vi "main.vi"() -> ()   [LabVIEW 2016]
uses:
  controls/Level2.ctl
panel:
  in  "BigCluster":T2
  in  "Cluster":T3
  in  "String":string
  in  "Boolean":bool
  in  "Numeric":dbl
  in  "Tab Control":enum32{"Page 1", "Page SubPanel"}(tab)
  in  "BigCluster":T2
  in  "Cluster":T3
  in  "String":string
  in  "Boolean":bool
  in  "Numeric":dbl
  in  "Panel Name":string
  in  "Refresh":bool
  in  "Listbox":i32(listbox)
  in  "OK":bool
  in  "Stop":bool
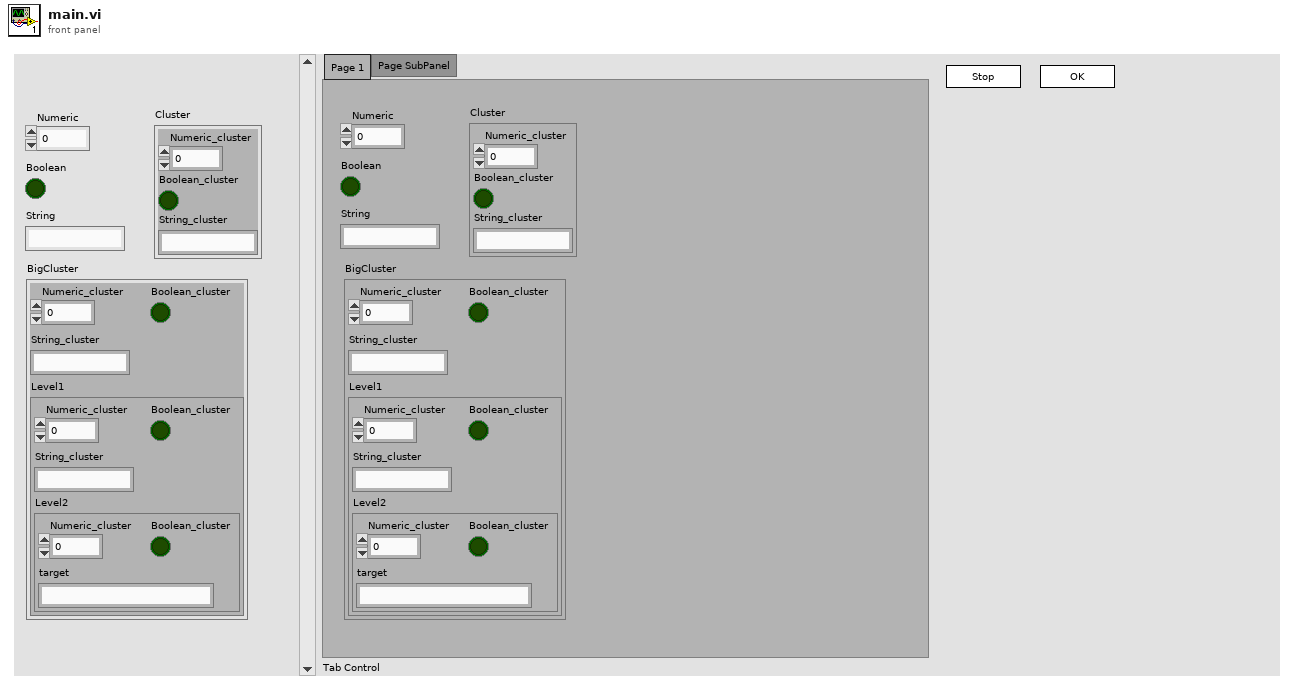
[diagram p1: front panel]
types:
  T1 = typedef "Level2.ctl" = cluster{"Numeric_cluster":dbl, "Boolean_cluster":bool, "target":string}
  T2 = cluster{"Numeric_cluster":dbl, "Boolean_cluster":bool, "String_cluster":string, "Level1":cluster{"Numeric_cluster":dbl, "Boolean_cluster":bool, "String_cluster":string, "Level2":T1}}
  T3 = cluster{"Numeric_cluster":dbl, "Boolean_cluster":bool, "String_cluster":string}
  T4 = enum32{"Invalid", "Standard", "Closed", "Hidden", "Minimized", "Maximized"}
  T5 = enum32{"invalid app kind", "Development System", "Run Time System", "Student Edition", "Embedded LabVIEW", "Evaluation", "Custom"}
  T6 = cluster{"Core":cluster{"Current VI Reference":refnum<vi>, "Close Panel on Exit?":bool}, "VI Name":string, "VI Ref":refnum<vi>, "Panel Folder Path":path}
  T7 = cluster{"Current VI Reference":refnum<vi>, "Close Panel on Exit?":bool}
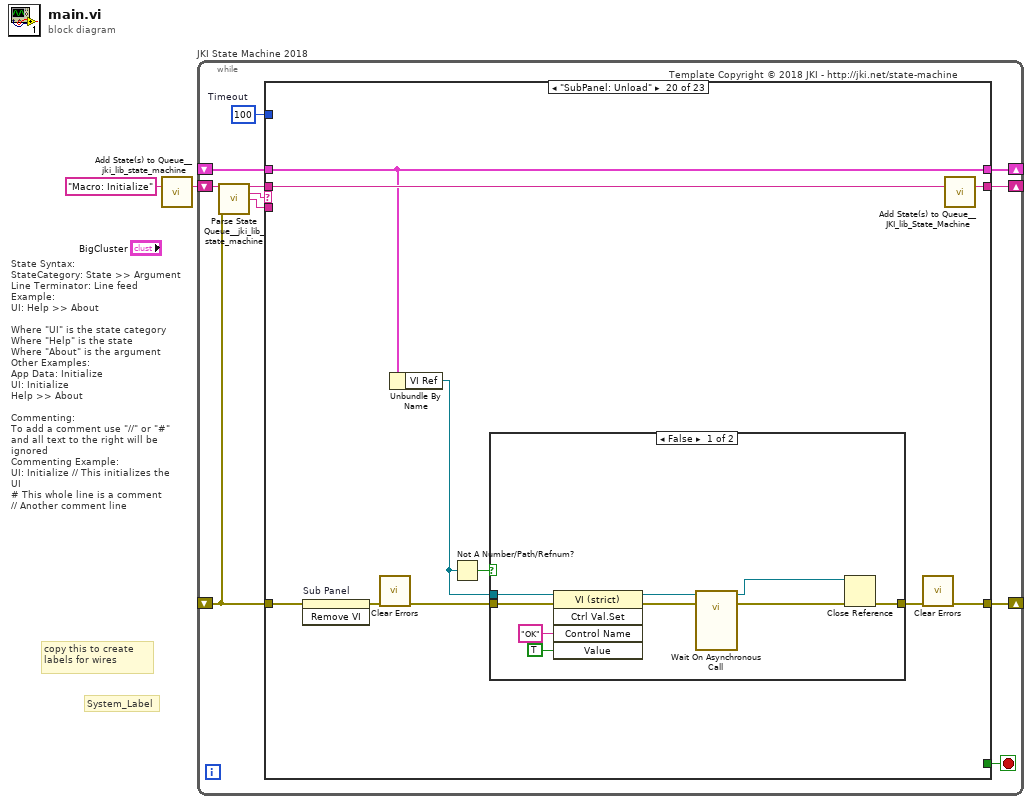
[diagram p0: block diagram]
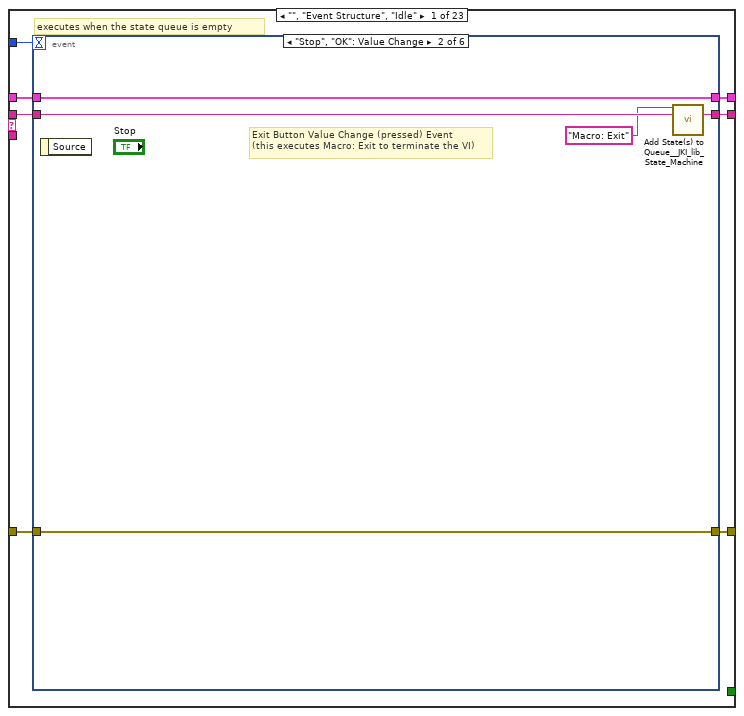
[diagram p2: hidden frame]
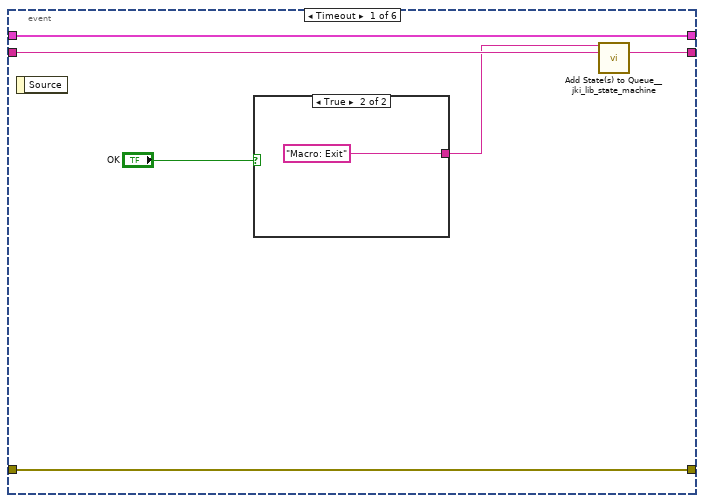
[diagram p3: hidden frame]
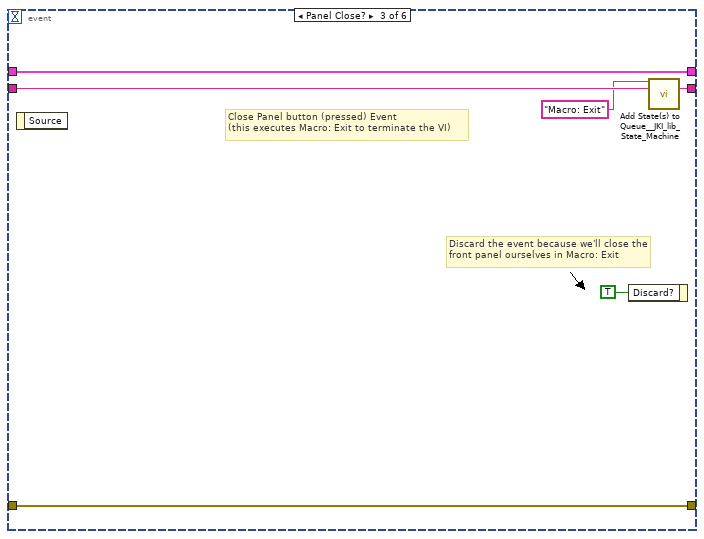
[diagram p5: hidden frame]
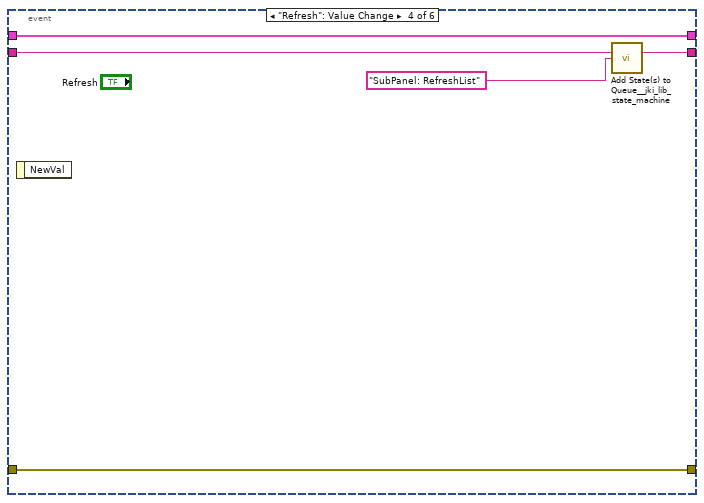
[diagram p6: hidden frame]
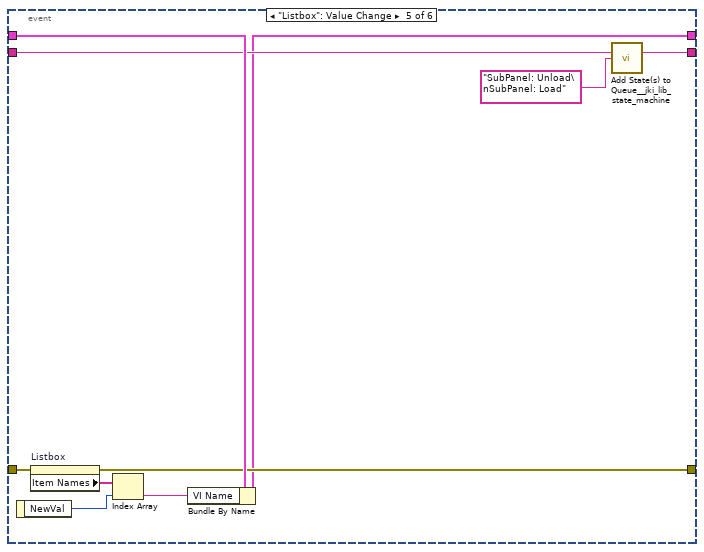
[diagram p7: hidden frame]
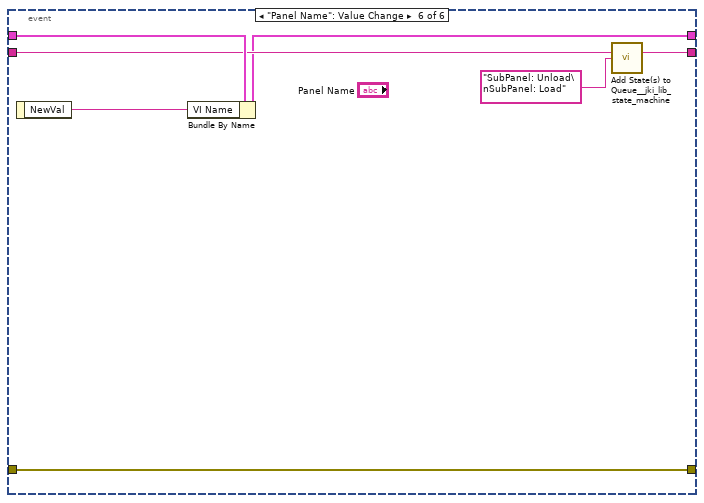
[diagram p8: hidden frame]
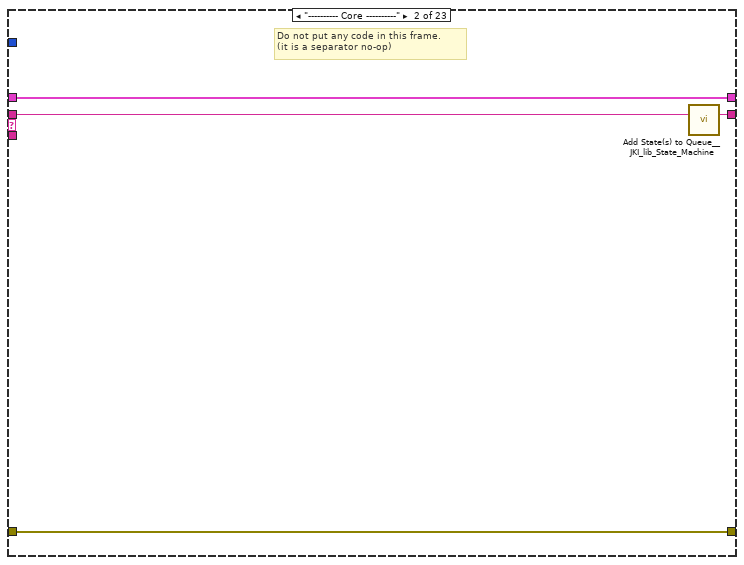
[diagram p9: hidden frame]
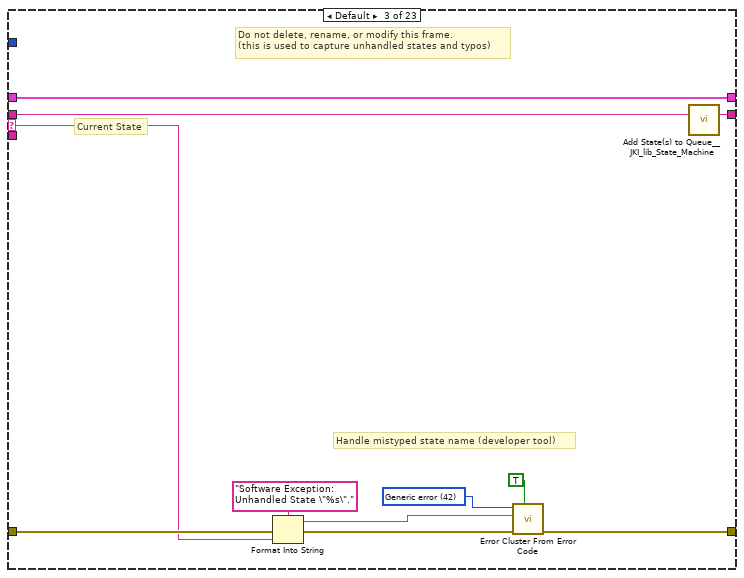
[diagram p10: hidden frame]
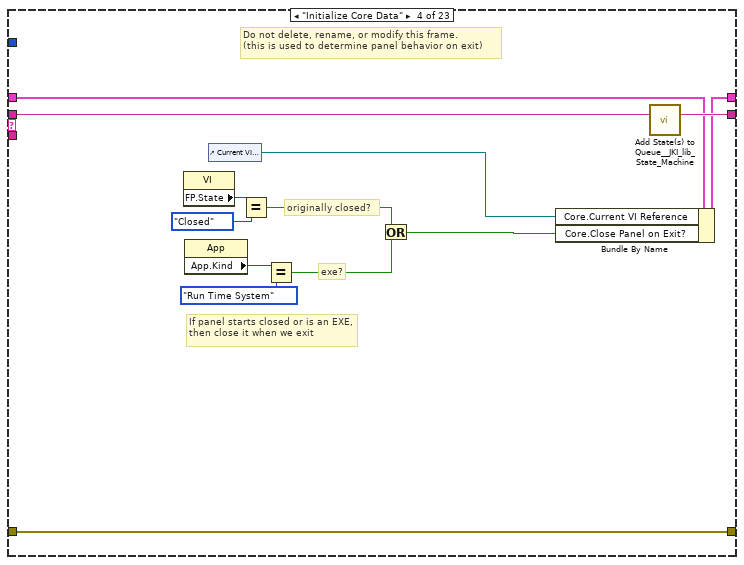
[diagram p11: hidden frame]
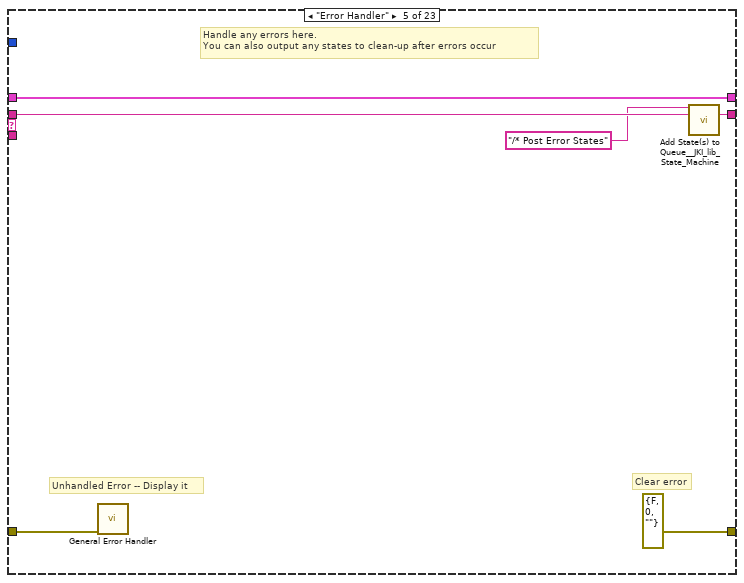
[diagram p12: hidden frame]
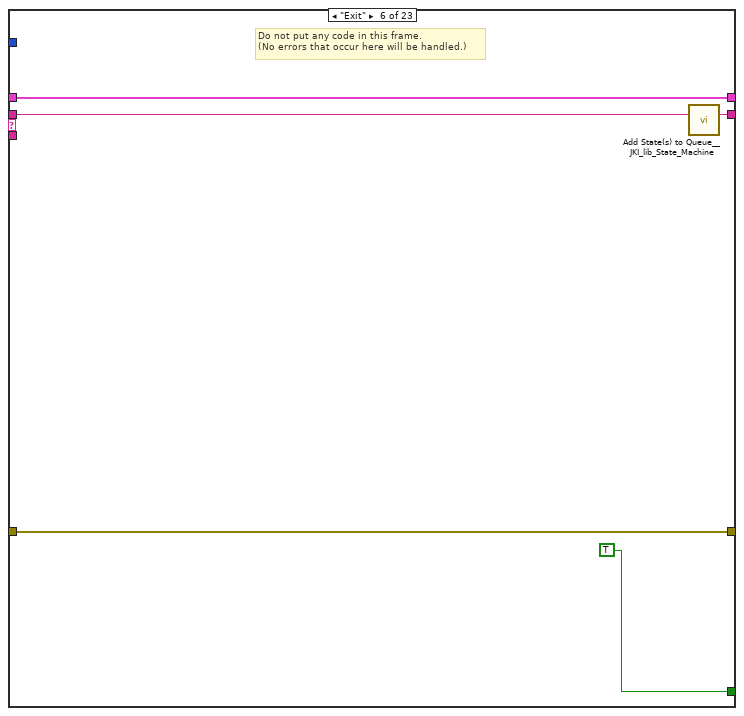
[diagram p13: hidden frame]
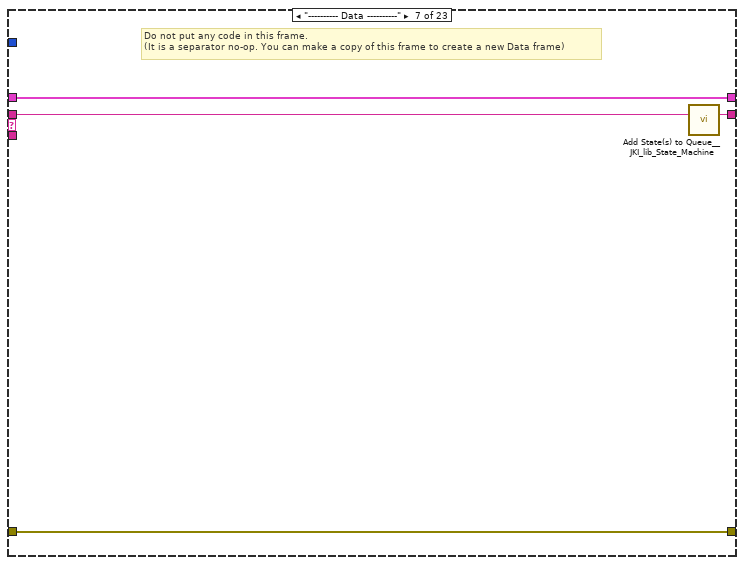
[diagram p14: hidden frame]
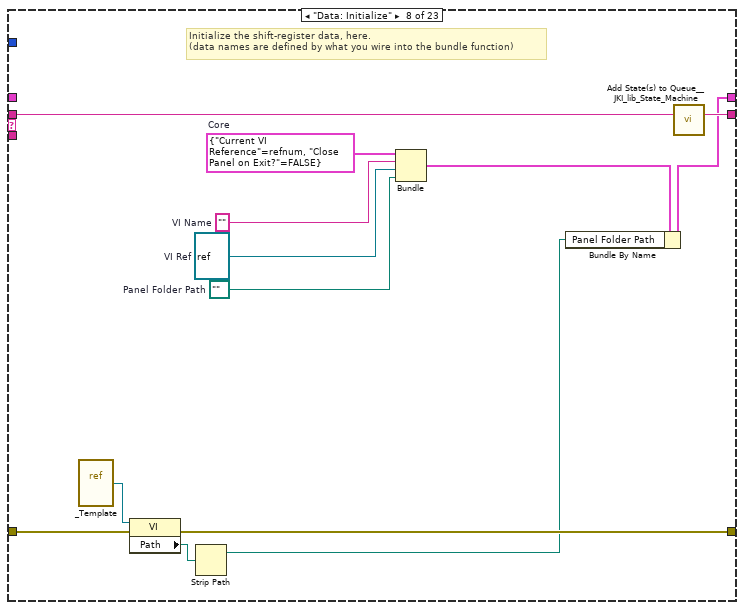
[diagram p15: hidden frame]
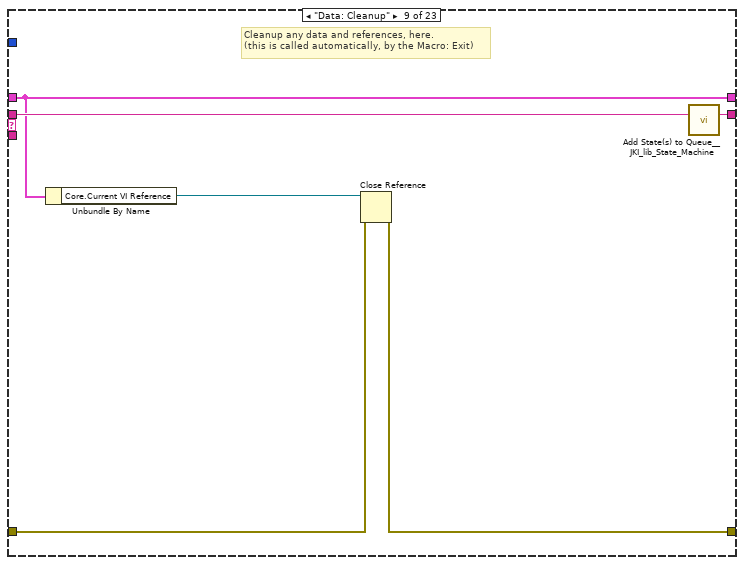
[diagram p16: hidden frame]
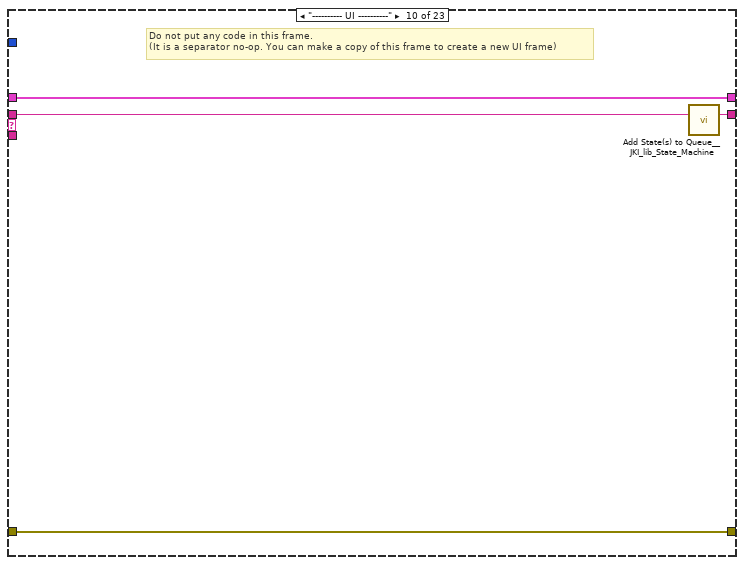
[diagram p17: hidden frame]
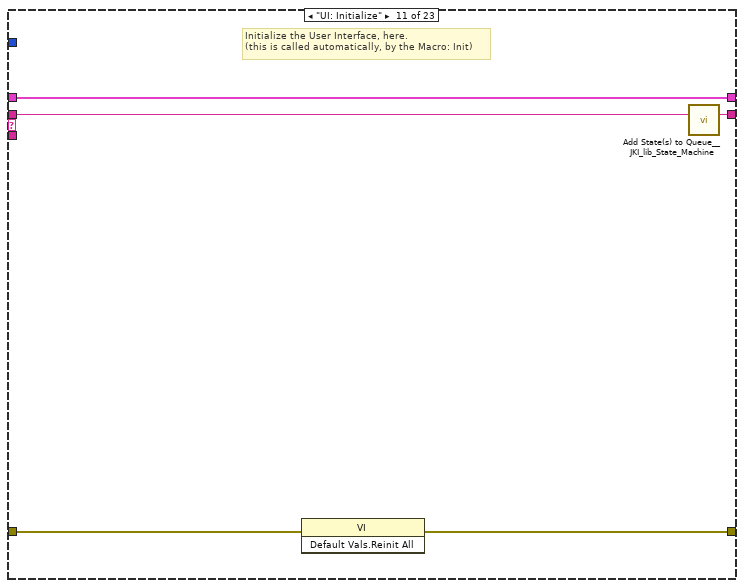
[diagram p18: hidden frame]
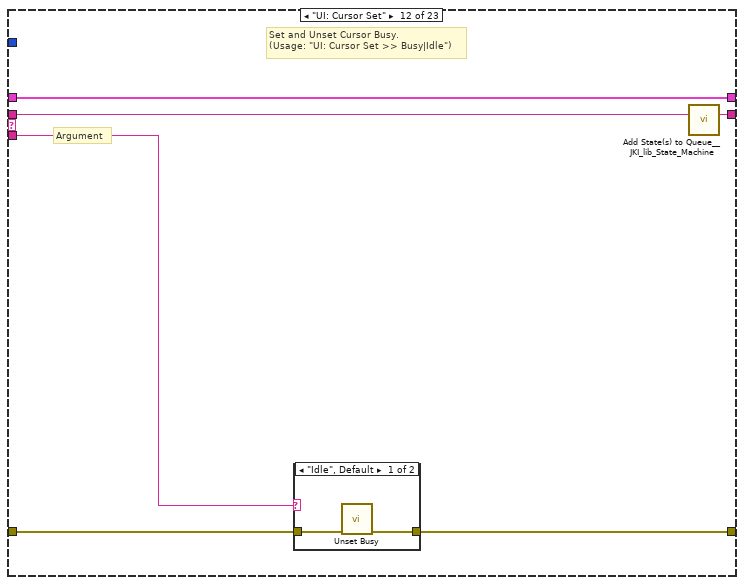
[diagram p19: hidden frame]
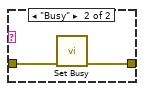
[diagram p20: hidden frame]
diagram:
  # "State Syntax:\nStateCategory: State >> Argument\nLine Terminator: Line feed\nExample:\nUI: Help >> About\n\nWhere \"UI\" is the state category\nWhere \"Help\" is the state\nWhere \"About\" is the argument\nOther Examples:\nApp Data: Initialize\nUI: Initialize\nHelp >> About\n\nCommenting:\nTo add a comment use \"//\" or \"#\" and all text to the right will be ignored\nCommenting Example:\nUI: Initialize // This initializes the UI\n# This whole line is a comment\n// Another comment line"
  # "copy this to create labels for wires"
  # "System_Label"
  n1 = call <vilib>:"Add State(s) to Queue__jki_lib_state_machine.vi"("State(s) in (\"\")"="Macro: Initialize") -> ("States Out"=w2:string)  [unwired: 14 in]
  n2 = while "JKI State Machine 2018" {
    shift-right: [w6] -> _
    shift-left: _ -> [w5]
    shift-right: [w9] -> _
    shift-left: _ -> [w3]
    shift-right: [w8] -> _
    shift-left: w2 -> [w10]
    stop <- w7 stop-if-true
    w4 = 100  # Timeout
    # "Template Copyright © 2018 JKI - http://jki.net/state-machine"
    n3 = call <vilib>:"Parse State Queue__jki_lib_state_machine.vi"("State Queue"=w10, "Error In (no error)"=w3) -> ("Remaining States"=w12:string, "Current State"=w13:string, "Arguments"=w11:string)  [unwired: 11 in]
    n4 = case shown="\"SubPanel: Unload\"" w13 {
      selector: w13 -> [_ _ w65 _ _ _ _ _ _ _ _ _ _ _ _ _ _ _ _ _ _ _ _]
      tunnel: w12 -> [w20 w64 w69 w88 w94 w99 w103 w116 w122 w126 w131 w137 w148 w217 w221 w226 w236 w240 w250 w260 w279 w307 w311]
      tunnel: w11 -> [_ _ _ _ _ _ _ _ _ _ _ w132 w142 _ _ _ _ _ _ _ _ _ _]
      tunnel: w5 -> [w18 w61 w67 w81 w91 w97 w100 _ w117 w123 w129 w135 w144 w215 w218 w223 w233 w237 w244 w257 w273 w304 w308]
      tunnel: [w17 w62 w71 w85 errorcluster {"status"=FALSE, "code"=0, "source"=""} ("error out") w96 w101 w108 w118 w124 w127 w133 w145 w214 w219 w224 w234 w238 w246 w251 w277 w305 w309] -> w9
      tunnel: w3 -> [w16 w62 w70 w85 w90 w96 w101 w109 w119 w124 w128 w134 w146 w214 w219 w224 w234 w238 w248 w253 w276 w305 w309]
      tunnel: [w19 w63 w68 w87 w93 w98 w102 w115 w121 w125 w130 w136 w147 w216 w220 w225 w235 w239 w249 w259 w278 w306 w310] -> w8
      tunnel: [_ _ _ _ _ TRUE _ _ _ _ _ _ _ _ _ _ _ _ _ _ _ _ _] -> w7
      tunnel: [w15 w61 w67 w86 w91 w97 w100 w110 w117 w123 w129 w135 w144 w215 w218 w223 w233 w237 w244 w257 w272 w304 w308] -> w6
      tunnel: w4 -> [w14 _ _ _ _ _ _ _ _ _ _ _ _ _ _ _ _ _ _ _ _ _ _]
      frame "", "Event Structure", "Idle" {
        # "executes when the state queue is empty"
        n5 = event shown="[1] \"Stop\", \"OK\": Value Change" {
          selector: _ -> [_ _ _ _ _ _]
          dyn-events: _ -> [_ _ _ _ _ _]
          timeout: w14 -> [_ _ _ _ _ _]
          tunnel: w20 -> [w26 w32 w38 w41 w52 w59]
          tunnel: [w25 w31 w37 w40 w51 w58] -> w19
          tunnel: w18 -> [w23 w29 w35 w42 w53 w60]
          tunnel: [w24 w30 w36 w43 w48 w56] -> w17
          tunnel: w16 -> [w24 w30 w36 w43 w49 w56]
          tunnel: [w23 w29 w35 w42 w45 w54] -> w15
          event Timeout {
            n6 = event-data() -> ()  [unwired: 1 in, 1 out]
            n7 = case shown="True" "OK" {
              tunnel: [_ "Macro: Exit"] -> w21
              frame False {
              }
              frame True {
              }
            }
            n8 = call <vilib>:"Add State(s) to Queue__jki_lib_state_machine.vi"("State(s) in Front (\"\")"=w21, "State(s) in (\"\")"=w26) -> ("States Out"=w25:string)  [unwired: 13 in]
          }
          event "Stop", "OK": Value Change {
            # "Exit Button Value Change (pressed) Event\n(this executes Macro: Exit to terminate the VI)"
            n9 = event-data() -> ()  [unwired: 1 in, 1 out]
            n10 = call <vilib>:"Add State(s) to Queue__JKI_lib_State_Machine.vi"("State(s) in Front (\"\")"="Macro: Exit", "State(s) in (\"\")"=w32) -> ("States Out"=w31:string)  [unwired: 13 in]
          }
          event Panel Close? {
            # "Discard the event because we'll close the front panel ourselves in Macro: Exit"
            # "Close Panel button (pressed) Event\n(this executes Macro: Exit to terminate the VI)"
            n11 = event-data() -> ()  [unwired: 1 in, 1 out]
            n12 = event-data("Discard?"=TRUE) -> ()  [unwired: 1 in, 1 out]
            n13 = call <vilib>:"Add State(s) to Queue__JKI_lib_State_Machine.vi"("State(s) in Front (\"\")"="Macro: Exit", "State(s) in (\"\")"=w38) -> ("States Out"=w37:string)  [unwired: 13 in]
          }
          event "Refresh": Value Change {
            n14 = event-data() -> ()  [unwired: 1 in, 1 out]
            n15 = call <vilib>:"Add State(s) to Queue__jki_lib_state_machine.vi"("State(s) in (\"\")"=w41, "State(s) at Back (\"\")"="SubPanel: RefreshList") -> ("States Out"=w40:string)  [unwired: 13 in]
          }
          event "Listbox": Value Change {
            n16 = event-data() -> ("NewVal"=w46:i32)  [unwired: 1 in]
            n17 = property on="Listbox" class="LstBox (strict)"(error in=w49) -> (error out=w48:errorcluster, "Item Names"=w47:string[])  [unwired: 1 in, 1 out]
            n18 = Index Array(array=w47, index=w46) -> (element=w44:string)
            n19 = Bundle By Name(cluster=w53, "VI Name"=w44) -> (w45:T6)
            n20 = call <vilib>:"Add State(s) to Queue__jki_lib_state_machine.vi"("State(s) in (\"\")"=w52, "State(s) at Back (\"\")"="SubPanel: Unload\nSubPanel: Load") -> ("States Out"=w51:string)  [unwired: 13 in]
          }
          event "Panel Name": Value Change {
            n21 = event-data() -> ("NewVal"=w55:string)  [unwired: 1 in]
            n22 = Bundle By Name(cluster=w60, "VI Name"=w55) -> (w54:T6)
            n23 = call <vilib>:"Add State(s) to Queue__jki_lib_state_machine.vi"("State(s) in (\"\")"=w59, "State(s) at Back (\"\")"="SubPanel: Unload\nSubPanel: Load") -> ("States Out"=w58:string)  [unwired: 13 in]
          }
        }
      }
      frame "---------- Core ----------" {
        # "Do not put any code in this frame.\n(it is a separator no-op)"
        n24 = call <vilib>:"Add State(s) to Queue__JKI_lib_State_Machine.vi"("State(s) in (\"\")"=w64) -> ("States Out"=w63:string)  [unwired: 14 in]
      }
      frame Default {
        w74 = 42 items=["No error", "Argument error", "Memory is full", "Out of zone", "End of file", "File already open", "Generic file I/O error", "File not found", "File permission error", "Disk is full", "Duplicate path", "Too many files open", "System feature not enabled", "Resource file not found", "Cannot add resource", "Resource not found", "Image not found", "Image memory error", "Pen does not exist", "Config type invalid", "Config token not found", "Config parse error", "Config memory error", "Bad external code format", "Bad external code offset", "External code not present", "Null window", "Destroy window error", "Null menu", "Print aborted", "Bad print record", "Print driver error", "Windows error during printing", "Memory error during printing", "Print dialog error", "Generic print error", "Invalid device refnum", "Device not found", "Device parameter error", "Device unit error", "Cannot open device", "Device call aborted", "Generic error", "Cancelled by user", "Object ID too low", "Object ID too high", "Object not in heap", "Unknown heap", "Unknown object (invalid DefProc)", "Unknown object (DefProc not in table)", "Message out of range", "Invalid (null) method", "Unknown message", "Manager call not supported", "Bad address", "Network operation in progress", "Network operation timed out", "Connection is busy", "Network attribute not supported", "Network error", "Address in use", "System out of memory", "Connection aborted", "Connection refused", "Not connected", "Already connected", "Connection closed", "Initialization error (interapplication manager)", "Bad occurrence", "Wait on unbound occurrence handler", "Occurrence queue overflow", "Datalog type conflict", "Unused", "Unrecognized type (interapplication manager)", "Memory corrupt", "Failed to make temporary DLL", "Old CIN version", "Drag socket not found", "Failed to load drop-object", "Failed to register OLE object", "Failed to release OLE object", "Format specifier type mismatch", "Unknown format specifier", "Too few format specifiers", "Too many format specifiers", "Scan failed", "Newer CIN version", "Error converting to variant", "Runtime menu error", "Password tampered", "Variant attribute not found", "Incompatible variant data type", "Event data is not available", "Event Store is not present", "Occurrence is not found", "Event Queue is not created", "Event info is not available", "Refnum passed is NULL", "Error retrieving Class GUID", "Error retrieving CoClass GUID", "Error retrieving TypeLib GUID.", "Bad built application magic bytes.", "Specific driver is different from the specific driver associated with the Logical Name.", "There is no session opened to the class driver.", "Max Error", "MAX - Error with config objects", "MAX - Error loading configuration", "MAX - Group not supported"]
        # "Current State"
        # "Do not delete, rename, or modify this frame.\n(this is used to capture unhandled states and typos)"
        # "Handle mistyped state name (developer tool)"
        n25 = Format Into String(format string="Software Exception: Unhandled State \"%s\"." ("message"), error in=w70, w65) -> (resulting string=w73:string, error out=w72:errorcluster)  [unwired: 1 in]
        n26 = call <vilib>:"Error Cluster From Error Code.vi"("show call chain? (False)"=TRUE, "error in (no error)"=w72, "error message (\"\")"=w73, "error code (0)"=w74) -> ("error out"=w71:errorcluster)  [unwired: 5 in]
        n27 = call <vilib>:"Add State(s) to Queue__JKI_lib_State_Machine.vi"("State(s) in (\"\")"=w69) -> ("States Out"=w68:string)  [unwired: 14 in]
      }
      frame "Initialize Core Data" {
        # "Do not delete, rename, or modify this frame.\n(this is used to determine panel behavior on exit)"
        # "originally closed?"
        # "exe?"
        # "If panel starts closed or is an EXE, then close it when we exit"
        n28 = property class="VI"() -> ("FP.State"=w78:T4)  [unwired: 2 in, 2 out]
        n29 = property class="App"() -> ("App.Kind"=w84:T5)  [unwired: 2 in, 2 out]
        n30 = control-ref of="Current VI Reference"() -> (w79:refnum<vi>)
        n31 = Equal?(x=w78, y=T4."Closed" ("Front Panel Window:State")) -> (x = y?=w76:bool)
        n32 = Equal?(x=w84, y=T5."Run Time System" ("Application:Kind")) -> (x = y?=w82:bool)
        n33 = Or(x=w76, y=w82) -> (x .or. y?=w80:bool)
        n34 = Bundle By Name(cluster=w81, "Core.Current VI Reference"=w79, "Core.Close Panel on Exit?"=w80) -> (w86:T6)
        n35 = call <vilib>:"Add State(s) to Queue__JKI_lib_State_Machine.vi"("State(s) in (\"\")"=w88) -> ("States Out"=w87:string)  [unwired: 14 in]
      }
      frame "Error Handler" {
        # "Unhandled Error -- Display it"
        # "Handle any errors here.\nYou can also output any states to clean-up after errors occur"
        # "Clear error"
        n36 = call <vilib>:"General Error Handler.vi"("error in (no error)"=w90) -> ()  [unwired: 10 in, 5 out]
        n37 = call <vilib>:"Add State(s) to Queue__JKI_lib_State_Machine.vi"("State(s) in Front (\"\")"="/* Post Error States", "State(s) in (\"\")"=w94) -> ("States Out"=w93:string)  [unwired: 13 in]
      }
      frame "Exit" {
        # "Do not put any code in this frame.\n(No errors that occur here will be handled.)"
        n38 = call <vilib>:"Add State(s) to Queue__JKI_lib_State_Machine.vi"("State(s) in (\"\")"=w99) -> ("States Out"=w98:string)  [unwired: 14 in]
      }
      frame "---------- Data ----------" {
        # "Do not put any code in this frame.\n(It is a separator no-op. You can make a copy of this frame to create a new Data frame)"
        n39 = call <vilib>:"Add State(s) to Queue__JKI_lib_State_Machine.vi"("State(s) in (\"\")"=w103) -> ("States Out"=w102:string)  [unwired: 14 in]
      }
      frame "Data: Initialize" {
        w104 = refnum<vi> refnum  # VI Ref
        w111 = path ""  # Panel Folder Path
        w112 = T7 {"Current VI Reference"=refnum, "Close Panel on Exit?"=FALSE}  # Core
        w113 = ""  # VI Name
        # "Initialize the shift-register data, here.\n(data names are defined by what you wire into the bundle function)"
        n40 = vi-ref "_Template.vi"() -> (w107:refnum<vi>)
        n41 = property class="VI"(reference=w107, error in=w109) -> (error out=w108:errorcluster, "Path"=w106:path)  [unwired: 1 out]
        n42 = Strip Path(path=w106) -> (stripped path=w105:path)  [unwired: 1 out]
        n43 = Bundle("Core"=w112, "VI Name"=w113, "VI Ref"=w104, "Panel Folder Path"=w111) -> (w114:T6)  [unwired: 1 in]
        n44 = Bundle By Name(cluster=w114, "Panel Folder Path"=w105) -> (w110:T6)
        n45 = call <vilib>:"Add State(s) to Queue__JKI_lib_State_Machine.vi"("State(s) in (\"\")"=w116) -> ("States Out"=w115:string)  [unwired: 14 in]
      }
      frame "Data: Cleanup" {
        # "Cleanup any data and references, here.\n(this is called automatically, by the Macro: Exit)"
        n46 = Unbundle By Name(w117) -> ("Core.Current VI Reference"=w120:refnum<vi>)
        n47 = Close Reference(reference=w120, error in (no error)=w119) -> (error out=w118:errorcluster)
        n48 = call <vilib>:"Add State(s) to Queue__JKI_lib_State_Machine.vi"("State(s) in (\"\")"=w122) -> ("States Out"=w121:string)  [unwired: 14 in]
      }
      frame "---------- UI ----------" {
        # "Do not put any code in this frame.\n(It is a separator no-op. You can make a copy of this frame to create a new UI frame)"
        n49 = call <vilib>:"Add State(s) to Queue__JKI_lib_State_Machine.vi"("State(s) in (\"\")"=w126) -> ("States Out"=w125:string)  [unwired: 14 in]
      }
      frame "UI: Initialize" {
        # "Initialize the User Interface, here.\n(this is called automatically, by the Macro: Init)"
        n50 = invoke class="VI" method="Default Vals.Reinit All"(error in=w128) -> (error out=w127:errorcluster)  [unwired: 2 in, 2 out]
        n51 = call <vilib>:"Add State(s) to Queue__JKI_lib_State_Machine.vi"("State(s) in (\"\")"=w131) -> ("States Out"=w130:string)  [unwired: 14 in]
      }
      frame "UI: Cursor Set" {
        # "Argument"
        # "Set and Unset Cursor Busy.\n(Usage: \"UI: Cursor Set >> Busy|Idle\")"
        n52 = case shown="\"Idle\", Default" w132 {
          tunnel: w134 -> [w139 w141]
          tunnel: [w138 w140] -> w133
          frame "Idle", Default {
            n53 = call <vilib>:"Unset Busy.vi"("error in (no error)"=w139) -> ("error out"=w138:errorcluster)  [unwired: 10 in]
          }
          frame "Busy" {
            n54 = call <vilib>:"Set Busy.vi"("error in (no error)"=w141) -> ("error out"=w140:errorcluster)  [unwired: 9 in, 1 out]
          }
        }
        n55 = call <vilib>:"Add State(s) to Queue__JKI_lib_State_Machine.vi"("State(s) in (\"\")"=w137) -> ("States Out"=w136:string)  [unwired: 14 in]
      }
      frame "UI: Front Panel State" {
        # "Argument"
        # "Set Front Panel Open or Closed\n(Usage: \"UI: Front Panel State >> Open|Close\")"
        n56 = Unbundle By Name(w144) -> ("Core.Current VI Reference"=w143:refnum<vi>)
        n57 = case shown="\"Close\", \"Closed\"" w142 {
          tunnel: w146 -> [w154 w169 w180 w193 w206]
          tunnel: [w156 w170 w182 w195 w208] -> w145
          tunnel: w143 -> [w155 w167 w181 w194 w207]
          frame "Open", "Standard", Default {
            w149 = T4."Standard" ("State")
            n58 = property class="VI"(reference=w155, error in=w154) -> (reference out=w152:refnum<vi>, error out=w153:errorcluster, "FP.State"=w151:T4)
            n59 = Not Equal?(x=w151, y=w149) -> (x != y?=w150:bool)
            n60 = case shown="True" w150 {
              tunnel: [w160 w162] -> w156
              tunnel: w153 -> [w159 w162]
              tunnel: w152 -> [w158 _]
              tunnel: w149 -> [w157 _]
              frame True {
                n61 = invoke class="VI" method="FP.Open"(reference=w158, error in=w159, "Activate"=TRUE, "State"=w157) -> (error out=w160:errorcluster)  [unwired: 1 in, 4 out]
              }
              frame False {
              }
            }
          }
          frame "Close", "Closed" {
            n62 = property class="VI"(reference=w167, error in=w169) -> (reference out=w166:refnum<vi>, error out=w168:errorcluster, "FP.State"=w164:T4)
            n63 = Not Equal?(x=w164, y=T4."Closed" ("Front Panel Window:State")) -> (x != y?=w163:bool)
            n64 = case shown="True" w163 {
              tunnel: [w171 w174] -> w170
              tunnel: w168 -> [w171 w173]
              tunnel: w166 -> [_ w172]
              frame False {
              }
              frame True {
                n65 = invoke class="VI" method="FP.Close"(reference=w172, error in=w173) -> (error out=w174:errorcluster)  [unwired: 1 in, 2 out]
              }
            }
          }
          frame "Hidden", "Hide" {
            w175 = T4."Hidden" ("State")
            n66 = property class="VI"(reference=w181, error in=w180) -> (reference out=w178:refnum<vi>, error out=w179:errorcluster, "FP.State"=w177:T4)
            n67 = Not Equal?(x=w177, y=w175) -> (x != y?=w176:bool)
            n68 = case shown="True" w176 {
              tunnel: [w186 w187] -> w182
              tunnel: w179 -> [w185 w187]
              tunnel: w178 -> [w184 _]
              tunnel: w175 -> [w183 _]
              frame True {
                n69 = invoke class="VI" method="FP.Open"(reference=w184, error in=w185, "State"=w183) -> (error out=w186:errorcluster)  [unwired: 2 in, 4 out]
              }
              frame False {
              }
            }
          }
          frame "Minimize", "Minimized" {
            w188 = T4."Minimized" ("State")
            n70 = property class="VI"(reference=w194, error in=w193) -> (reference out=w191:refnum<vi>, error out=w192:errorcluster, "FP.State"=w190:T4)
            n71 = Not Equal?(x=w190, y=w188) -> (x != y?=w189:bool)
            n72 = case shown="True" w189 {
              tunnel: [w199 w200] -> w195
              tunnel: w192 -> [w198 w200]
              tunnel: w191 -> [w197 _]
              tunnel: w188 -> [w196 _]
              frame True {
                n73 = invoke class="VI" method="FP.Open"(reference=w197, error in=w198, "State"=w196) -> (error out=w199:errorcluster)  [unwired: 2 in, 4 out]
              }
              frame False {
              }
            }
          }
          frame "Maximize", "Maximized" {
            w201 = T4."Maximized" ("State")
            n74 = property class="VI"(reference=w207, error in=w206) -> (reference out=w204:refnum<vi>, error out=w205:errorcluster, "FP.State"=w203:T4)
            n75 = Not Equal?(x=w203, y=w201) -> (x != y?=w202:bool)
            n76 = case shown="True" w202 {
              tunnel: [w212 w213] -> w208
              tunnel: w205 -> [w211 w213]
              tunnel: w204 -> [w210 _]
              tunnel: w201 -> [w209 _]
              frame True {
                n77 = invoke class="VI" method="FP.Open"(reference=w210, error in=w211, "State"=w209) -> (error out=w212:errorcluster)  [unwired: 2 in, 4 out]
              }
              frame False {
              }
            }
          }
        }
        n78 = call <vilib>:"Add State(s) to Queue__JKI_lib_State_Machine.vi"("State(s) in (\"\")"=w148) -> ("States Out"=w147:string)  [unwired: 14 in]
      }
      frame "UI: Update" {
        n79 = call <vilib>:"Add State(s) to Queue__JKI_lib_State_Machine.vi"("State(s) in (\"\")"=w217) -> ("States Out"=w216:string)  [unwired: 14 in]
      }
      frame "---------- Macro ----------" {
        # "Do not put any code in this frame.\n(It is a separator no-op. You can make a copy of this frame to create a new Macro frame)"
        n80 = call <vilib>:"Add State(s) to Queue__JKI_lib_State_Machine.vi"("State(s) in (\"\")"=w221) -> ("States Out"=w220:string)  [unwired: 14 in]
      }
      frame "Macro: Initialize" {
        w222 = "Data: Initialize\nInitialize Core Data\nUI: Initialize\nUI: Front Panel State >> Open\n# Custom States\nSubPanel: RefreshList"  # Data: Initialize Initialize Core Data UI: Initialize UI: Front Panel State >> Open # Custom States SubPanel: RefreshList
        # "Initialization Macro\n(This is called once, when the VI starts)"
        n81 = call <vilib>:"Add State(s) to Queue__JKI_lib_State_Machine.vi"("State(s) in Front (\"\")"=w222, "State(s) in (\"\")"=w226) -> ("States Out"=w225:string)  [unwired: 13 in]
      }
      frame "Macro: Exit" {
        # "Exit Macro\n(This is called once, when the VI exits)"
        n82 = Unbundle By Name(w233) -> ("Core.Close Panel on Exit?"=w232:bool)
        n83 = Select(t="UI: Front Panel State >> Close", s=w232, f="") -> (s? t:f=w229:string)
        n84 = call <vilib>:"Add State(s) to Queue__JKI_lib_State_Machine.vi"("State(s) in (\"\")"=w229, "State(s) at Back (\"\")"="SubPanel: Unload\nData: Cleanup\nExit") -> ("States Out"=w227:string)  [unwired: 13 in]
        n85 = call <vilib>:"Add State(s) to Queue__JKI_lib_State_Machine.vi"("State(s) in Front (\"\")"=w227, "State(s) in (\"\")"=w236) -> ("States Out"=w235:string)  [unwired: 13 in]
      }
      frame "---------- SubPanel ----------" {
        # "Template Separator\n(You can make a copy of, or modify, this frame)"
        n86 = call <vilib>:"Add State(s) to Queue__JKI_lib_State_Machine.vi"("State(s) in (\"\")"=w240) -> ("States Out"=w239:string)  [unwired: 14 in]
      }
      frame "SubPanel: RefreshList" {
        n87 = Unbundle By Name(w244) -> ("Panel Folder Path"=w243:path)
        n88 = List Folder(path=w243, pattern="*.vi", error in=w248) -> (filenames=w245:string[], error out=w247:errorcluster)  [unwired: 1 in, 2 out]
        n89 = property on="Listbox" class="LstBox (strict)"(error in=w247, "Item Names"=w245, "Value"=-1 ("Listbox")) -> (error out=w246:errorcluster)  [unwired: 1 in, 1 out]
        n90 = call <vilib>:"Add State(s) to Queue__JKI_lib_State_Machine.vi"("State(s) in (\"\")"=w250) -> ("States Out"=w249:string)  [unwired: 14 in]
      }
      frame "SubPanel: Unload" {
        n91 = invoke on="Sub Panel" class="SubPnl" method="Remove VI"(error in=w253) -> (error out=w258:errorcluster)  [unwired: 2 in, 2 out]
        n92 = call <vilib>:"Clear Errors.vi"("error in (no error)"=w258) -> ("error out"=w252:errorcluster)  [unwired: 5 in, 1 out]
        n93 = Unbundle By Name(w257) -> ("VI Ref"=w256:refnum<vi>)
        n94 = Not A Number/Path/Refnum?(number/path/refnum=w256) -> (NaN/Path/Refnum?=w255:bool)
        n95 = case shown="False" w255 {
          tunnel: w252 -> [w269 w270]
          tunnel: [w265 w270] -> w254
          tunnel: w256 -> [w266 _]
          frame False {
            n96 = invoke class="VI (strict)" method="Ctrl Val.Set"(reference=w266, error in=w269, "Control Name"="OK", "Value"=TRUE) -> (reference out=w262:refnum<vi>, error out=w264:errorcluster)  [unwired: 1 in, 3 out]
            n97 = call-by-ref "Wait On Asynchronous Call"(reference=w262, error in=w264) -> (reference out=w261:refnum<vi>, error out=w263:errorcluster)  [unwired: 12 in]
            n98 = Close Reference(reference=w261, error in (no error)=w263) -> (error out=w265:errorcluster)
          }
          frame True {
          }
        }
        n99 = call <vilib>:"Clear Errors.vi"("error in (no error)"=w254) -> ("error out"=w251:errorcluster)  [unwired: 5 in, 1 out]
        n100 = call <vilib>:"Add State(s) to Queue__JKI_lib_State_Machine.vi"("State(s) in (\"\")"=w260) -> ("States Out"=w259:string)  [unwired: 14 in]
      }
      frame "SubPanel: Load" {
        n101 = Unbundle By Name(w273) -> ("VI Ref"=w271:refnum<vi>, "Panel Folder Path"=w275:path, "VI Name"=w274:string)
        n102 = case shown="Default" w274 {
          selector: w274 -> [_ w291]
          tunnel: [w281 w287] -> w277
          tunnel: w276 -> [w281 w286]
          tunnel: w275 -> [_ w292]
          tunnel: w273 -> [w280 w290]
          tunnel: [w280 w289] -> w272
          tunnel: w271 -> [_ w282]
          frame "" {
          }
          frame Default {
            n103 = Build Path(base path=w292, name or relative path=w291) -> (appended path=w284:path)
            n104 = File/Directory Info(path=w284, error in=w286) -> (path out=w283:path, error out=w285:errorcluster)  [unwired: 5 out]
            n105 = case shown="No Error" w285 {
              selector: w285 -> [w300 w303]
              tunnel: [w294 _] -> w288
              tunnel: [w296 w302] -> w287
              tunnel: w283 -> [w299 _]
              tunnel: w282 -> [w298 _]
              frame No Error {
                n106 = Open VI Reference(type specifier VI Refnum (for type only)=w298, vi path=w299, options=256, error in (no error)=w300) -> (vi reference=w295:refnum<vi>, error out=w301:errorcluster)  [unwired: 2 in]
                n107 = invoke on="Sub Panel" class="SubPnl" method="Insert VI"(error in=w301, "VI Ref"=w295) -> (error out=w297:errorcluster)  [unwired: 2 in, 3 out]
                n108 = call-by-ref "Start Asynchronous Call"(reference=w295, error in=w297) -> (reference out=w294:refnum<vi>, error out=w296:errorcluster)  [unwired: 12 in]
              }
              frame Error {
                n109 = call <vilib>:"Clear Errors.vi"("error in (no error)"=w303) -> ("error out"=w302:errorcluster)  [unwired: 5 in, 1 out]
              }
            }
            n110 = Bundle By Name(cluster=w290, "VI Ref"=w288) -> (w289:T6)
          }
        }
        n111 = call <vilib>:"Add State(s) to Queue__JKI_lib_State_Machine.vi"("State(s) in (\"\")"=w279) -> ("States Out"=w278:string)  [unwired: 14 in]
      }
      frame "---------- New Category ----------" {
        # "Template Separator\n(You can make a copy of, or modify, this frame)"
        n112 = call <vilib>:"Add State(s) to Queue__JKI_lib_State_Machine.vi"("State(s) in (\"\")"=w307) -> ("States Out"=w306:string)  [unwired: 14 in]
      }
      frame "New Category: 2" {
        # "Your code here.\n(You can make a copy of, or modify, this frame)"
        n113 = call <vilib>:"Add State(s) to Queue__JKI_lib_State_Machine.vi"("State(s) in (\"\")"=w311) -> ("States Out"=w310:string)  [unwired: 14 in]
      }
    }
  }
